vi "Create All Message Queues.vi"(8 "error in (no error)":errorcluster) -> (0 "error out":errorcluster, 3 "Message Queues out":T1)   [LabVIEW 2015, in "Message Queue.lvlib"]
doc: "This VI creates and initializes all the message queues for your application. If your application requires more than one message queue, right-click the \"Message Queues\" constant above and select Open Type Def. Add the new Message Queue(s) to the type definition, then initialize them in this VI."
uses:
  Message Queue.lvlib
  All Message Queues.ctl
  Message Cluster.ctl
  Enqueue Message (Single).vi
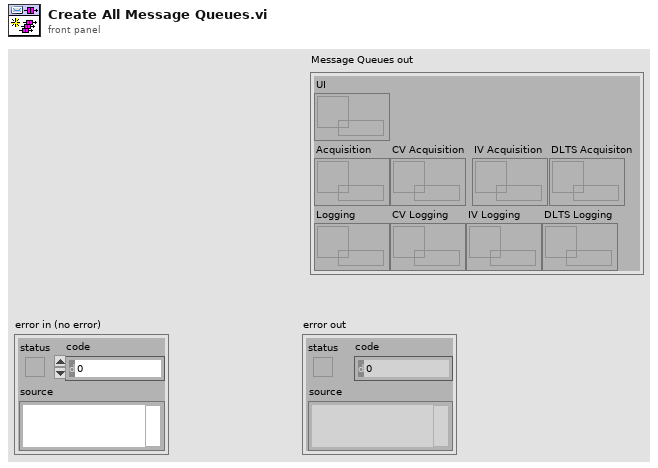
[diagram p1: front panel]
types:
  T1 = typedef "Message Queue.lvlib/All Message Queues.ctl" = cluster{"UI":refnum<queue>, "CV Acquisition":refnum<queue>, "CV Logging":refnum<queue>, "IV Acquisition":refnum<queue>, "IV Logging":refnum<queue>, "DLTS Acquisiton":refnum<queue>, "DLTS Logging":refnum<queue>, "Acquisition":refnum<queue>, "Logging":refnum<queue>}
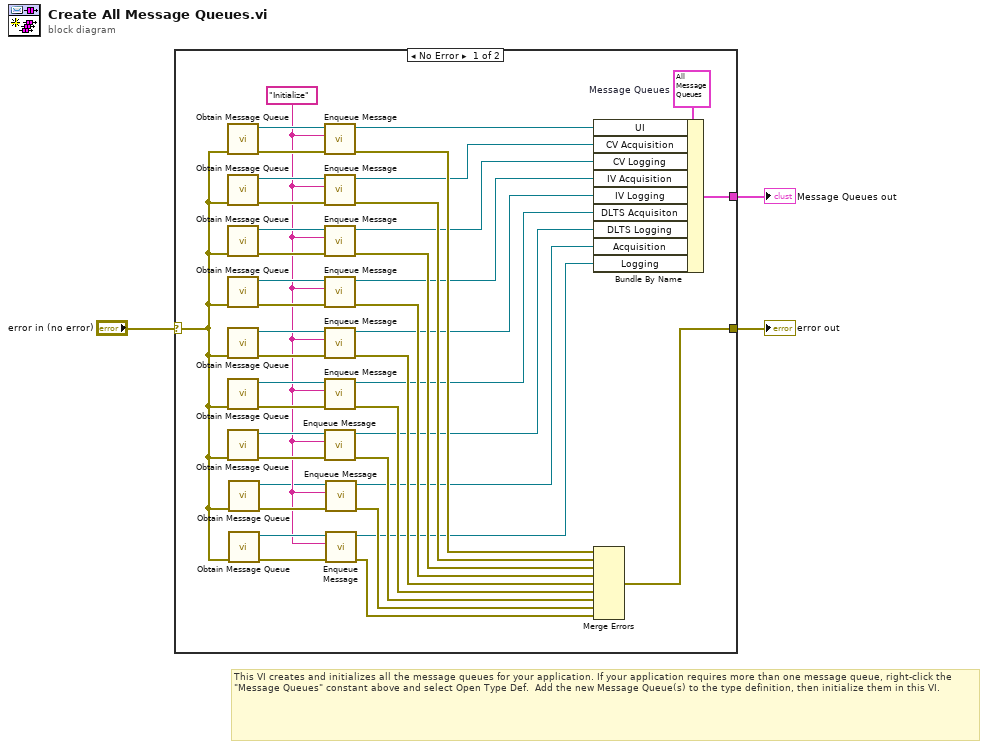
[diagram p0: block diagram]
diagram:
  # "This VI creates and initializes all the message queues for your application. If your application requires more than one message queue, right-click the \"Message Queues\" constant above and select Open Type Def.  Add the new Message Queue(s) to the type definition, then initialize them in this VI."
  n1 = case shown="No Error" "error in (no error)" {
    selector: "error in (no error)" -> [w15 w45]
    tunnel: [w34 w45] -> w3
    tunnel: [w42 _] -> w2
    frame No Error {
      w16 = "Initialize" ("Message")
      w43 = T1 {"UI"=refnum, "CV Acquisition"=refnum, "CV Logging"=refnum, "IV Acquisition"=refnum, "IV Logging"=refnum, "DLTS Acquisiton"=refnum, "DLTS Logging"=refnum, "Acquisition"=refnum, "Logging"=refnum}  # Message Queues
      n2 = call "Obtain Message Queue.vi"("error in (no error)"=w15) -> ("error out"=w41:errorcluster, "Message Queue"=w40:refnum<queue>)  [unwired: 9 in]
      n3 = call "Obtain Message Queue.vi"("error in (no error)"=w15) -> ("error out"=w38:errorcluster, "Message Queue"=w39:refnum<queue>)  [unwired: 9 in]
      n4 = call "Obtain Message Queue.vi"("error in (no error)"=w15) -> ("error out"=w37:errorcluster, "Message Queue"=w36:refnum<queue>)  [unwired: 9 in]
      n5 = call "Obtain Message Queue.vi"("error in (no error)"=w15) -> ("error out"=w28:errorcluster, "Message Queue"=w27:refnum<queue>)  [unwired: 9 in]
      n6 = call "Obtain Message Queue.vi"("error in (no error)"=w15) -> ("error out"=w29:errorcluster, "Message Queue"=w26:refnum<queue>)  [unwired: 9 in]
      n7 = call "Obtain Message Queue.vi"("error in (no error)"=w15) -> ("error out"=w30:errorcluster, "Message Queue"=w25:refnum<queue>)  [unwired: 9 in]
      n8 = call "Obtain Message Queue.vi"("error in (no error)"=w15) -> ("error out"=w31:errorcluster, "Message Queue"=w24:refnum<queue>)  [unwired: 9 in]
      n9 = call "Obtain Message Queue.vi"("error in (no error)"=w15) -> ("error out"=w18:errorcluster, "Message Queue"=w14:refnum<queue>)  [unwired: 9 in]
      n10 = call "Obtain Message Queue.vi"("error in (no error)"=w15) -> ("error out"=w17:errorcluster, "Message Queue"=w19:refnum<queue>)  [unwired: 9 in]
      n11 = call-poly "Enqueue Message.vi"("error in (no error)"=w41, "Message"=w16, "Message Queue"=w40) -> ("error out"=w44:errorcluster, "dup Message Queue"=w35:refnum<queue>)  [unwired: 7 in]
      n12 = call-poly "Enqueue Message.vi"("error in (no error)"=w38, "Message"=w16, "Message Queue"=w39) -> ("error out"=w33:errorcluster, "dup Message Queue"=w11:refnum<queue>)  [unwired: 7 in]
      n13 = call-poly "Enqueue Message.vi"("error in (no error)"=w37, "Message"=w16, "Message Queue"=w36) -> ("error out"=w32:errorcluster, "dup Message Queue"=w10:refnum<queue>)  [unwired: 7 in]
      n14 = call-poly "Enqueue Message.vi"("error in (no error)"=w28, "Message"=w16, "Message Queue"=w27) -> ("error out"=w23:errorcluster, "dup Message Queue"=w9:refnum<queue>)  [unwired: 7 in]
      n15 = call-poly "Enqueue Message.vi"("error in (no error)"=w29, "Message"=w16, "Message Queue"=w26) -> ("error out"=w22:errorcluster, "dup Message Queue"=w8:refnum<queue>)  [unwired: 7 in]
      n16 = call-poly "Enqueue Message.vi"("error in (no error)"=w30, "Message"=w16, "Message Queue"=w25) -> ("error out"=w21:errorcluster, "dup Message Queue"=w7:refnum<queue>)  [unwired: 7 in]
      n17 = call-poly "Enqueue Message.vi"("error in (no error)"=w31, "Message"=w16, "Message Queue"=w24) -> ("error out"=w20:errorcluster, "dup Message Queue"=w6:refnum<queue>)  [unwired: 7 in]
      n18 = call-poly "Enqueue Message.vi"("error in (no error)"=w18, "Message"=w16, "Message Queue"=w14) -> ("error out"=w12:errorcluster, "dup Message Queue"=w5:refnum<queue>)  [unwired: 7 in]
      n19 = call-poly "Enqueue Message.vi"("error in (no error)"=w17, "Message"=w16, "Message Queue"=w19) -> ("error out"=w13:errorcluster, "dup Message Queue"=w4:refnum<queue>)  [unwired: 7 in]
      n20 = Bundle By Name(cluster=w43, "UI"=w35, "CV Acquisition"=w11, "CV Logging"=w10, "IV Acquisition"=w9, "IV Logging"=w8, "DLTS Acquisiton"=w7, "DLTS Logging"=w6, "Acquisition"=w5, "Logging"=w4) -> (w42:T1)
      n21 = Merge Errors(w44, w33, w32, w23, w22, w21, w20, w12, w13) -> (w34:errorcluster)
    }
    frame Error {
    }
  }
  "Message Queues out" <- w2
  "error out" <- w3
